vi "Stop Core.vi"(10 "final error code":i32, 11 "IViewModel in":refnum<class "IViewModel.lvclass">) -> (3 "IViewModel out":refnum<class "IViewModel.lvclass">)   [LabVIEW 2017, in "IViewModel.lvlib" / "IViewModel.lvclass"]
doc: "(<B>Filename</B>: Actor Framework.lvlib:Actor.lvclass:Stop Core.vi)\n\nDefines what the actor does before it stops. Use the <B>final error code</B> input to determine whether the actor shut down in response to an error.\n\nBy default, this method does nothing. A descendant class may override it to define behavior, such as shutting down any processes the actor initiated in its override of the Actor Core method.\n\n<License>\nCopyright © 2017 Composed Systems, LLC | All rights reserved\nwww.composed.io\n\nAuthor: Ethan Stern <ethan.stern@composed.io>\n\nThis software is provided \"AS IS\" WITHOUT WARRANTIES, either express or implied, AND IS FOR EDUCATIONAL PURPOSES ONLY.\n</License>"
uses:
  IViewModel.lvclass
  IViewModel.lvclass/IViewModel.ctl
  <vilib>/ActorFramework/Message Enqueuer/Message Enqueuer.lvclass/Message Enqueuer.ctl
  gpm_packages/@cs/event-logger/Source/Composed Log/Log Sink/Log Level.ctl
  gpm_packages/@cs/event-logger/Source/Composed Log/Global Application Log/Message Log Worker.vi
  <vilib>/ActorFramework/Message Enqueuer/Enqueue.vi
  gpm_packages/@cs/event-logger/Source/Composed Log/Global Application Log/Invalid Reference Error.vi
  <vilib>/ActorFramework/Stop Msg/Stop Msg.lvclass
  C:/Program Files (x86)/National Instruments/LabVIEW 2017/vi.lib/ActorFramework/Message/Message.lvclass
  <vilib>/ActorFramework/Message Priority Queue/Priority Enqueue.vi
  gpm_packages/@cs/event-logger/Source/Composed Log/Global Application Log/Get Worker Queue.vi
  IViewManager/IViewManager/IViewManager.lvclass
  gpm_packages/@cs/event-logger/Source/Composed Log/LoggerReference/LoggerReference.lvclass
  IViewable/ProtectedSubpanel/ProtectedSubpanel.lvclass
  gpm_packages/@cs/event-logger/Source/Composed Log/Composed Log.lvlib
  gpm_packages/@cs/event-logger/Source/Composed Log/Log Sink/Log Sink.lvclass
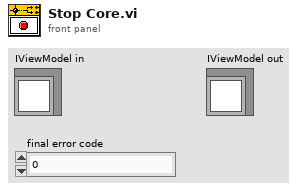
[diagram p1: front panel]
types:
  T1 = typedef "Composed Log.lvlib/Log Sink.lvclass/Log Level.ctl" = enum16{"Debug", "Info", "Warning", "Error", "Critical"}
  T2 = typedef "IViewable.lvlib/ProtectedSubpanel.lvclass/Protected Subpanel Reference.ctl" = refnum<data-value>
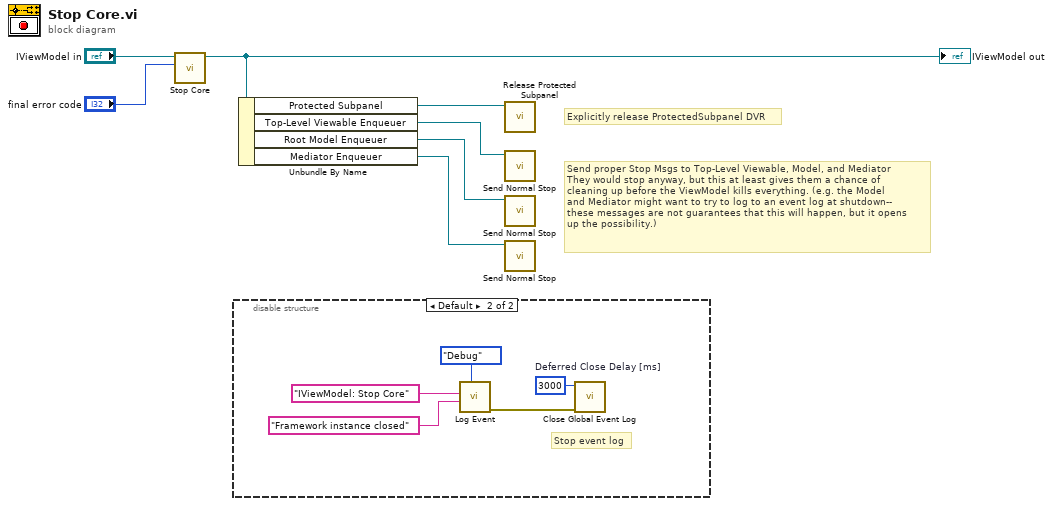
[diagram p0: block diagram]
diagram:
  # "Explicitly release ProtectedSubpanel DVR"
  # "Send proper Stop Msgs to Top-Level Viewable, Model, and Mediator\nThey would stop anyway, but this at least gives them a chance of\ncleaning up before the ViewModel kills everything. (e.g. the Model\nand Mediator might want to try to log to an event log at shutdown--\nthese messages are not guarantees that this will happen, but it opens\nup the possibility.)"
  n1 = call-parent "Stop Core.vi"("final error code"="final error code", "IViewManager in"="IViewModel in") -> ("IViewManager out"=w1:refnum<class "IViewModel.lvclass">)  [unwired: 9 in]
  "IViewModel out" <- w1
  n2 = disable-structure shown="Default" {
    frame condition #0 {
    }
    frame condition #1 (active) {
      w10 = u32 3000  # Deferred Close Delay [ms]
      # "Stop event log"
      n3 = call "Log Event.vi"("Event Level"=Log_Level."Debug", "Data To Log"="Framework instance closed", "SourceID"="IViewModel: Stop Core") -> ("error out"=w12:errorcluster)  [unwired: 7 in, 1 out]
      n4 = call "Close Global Event Log.vi"("error in (no error)"=w12, "Deferred Close Time (0 ms)"=w10) -> ()  [unwired: 9 in, 1 out]
    }
  }
  n5 = Unbundle By Name(w1) -> ("Protected Subpanel"=w2:T2, "Top-Level Viewable Enqueuer"=w3:refnum<class "Message Enqueuer.lvclass">, "Root Model Enqueuer"=w5:refnum<class "Message Enqueuer.lvclass">, "Mediator Enqueuer"=w4:refnum<class "Message Enqueuer.lvclass">)
  n6 = call "Release Protected Subpanel.vi"("Protected Subpanel"=w2) -> ()  [unwired: 10 in, 1 out]
  n7 = call <vilib>:"Send Normal Stop.vi"("Message Enqueuer"=w3) -> ()  [unwired: 10 in, 1 out]
  n8 = call <vilib>:"Send Normal Stop.vi"("Message Enqueuer"=w5) -> ()  [unwired: 10 in, 1 out]
  n9 = call <vilib>:"Send Normal Stop.vi"("Message Enqueuer"=w4) -> ()  [unwired: 10 in, 1 out]
